vi "Actor Core.vi"(8 "error in":errorcluster, 11 "Display Panel V3 in":refnum<class "Display Panel V3.lvclass">) -> (0 "error out":errorcluster, 3 "Actor out":refnum<class "Actor.lvclass">)   [LabVIEW 2014, in "Display Panel.lvlib" / "Display Panel V3.lvclass"]
doc: "(<B>Filename</B>: Actor Framework.lvlib:Actor.lvclass:Actor Core.vi)\n\nReceives messages to the actor, reacts to them, and initiates any error handling that may shut the actor down.\n\nDescendant classes may override this VI to append parallel tasks for the actor to complete while it handles messages. Overrides use the Call Parent Method node."
uses:
  Display Panel V3.lvclass
  <vilib>/ActorFramework/Actor/Actor.lvclass
  Controls/Numeric Indicator.ctl
  <vilib>/ActorFramework/Actor/Actor.lvclass/Actor.ctl
  <vilib>/ActorFramework/Message Enqueuer/Message Enqueuer.lvclass/Message Enqueuer.ctl
  <vilib>/ActorFramework/Stop Msg/Stop Msg.lvclass/Stop Msg.ctl
  <vilib>/ActorFramework/Message Enqueuer/Init from Existing Queue.vi
  <vilib>/ActorFramework/Message Enqueuer/Enqueue Critical.vi
  <vilib>/express/express shared/transition.llb/Dynamic To Waveform Array.vi
  <vilib>/ActorFramework/Message Priority Queue/Priority Enqueue.vi
  <vilib>/ActorFramework/Message Enqueuer/Message Enqueuer.lvclass
  <vilib>/express/express signal manip/GetorSetDDTAttributes/Get DDT Attributes/Get DDT Properties.xnode
  <vilib>/ActorFramework/Stop Msg/Stop Msg.lvclass
  Generic Instrument/Generic Instrument.lvclass
panel:
  out "String":string
  out "Card #":dbl
  out "Numeric Control":i32
  in  "Waveform Chart":dynamicdata(graph)
  out "Array":T1[](array[typedef])
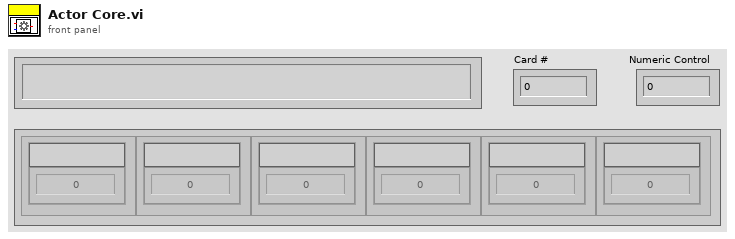
[diagram p1: front panel]
types:
  T1 = typedef "Numeric Indicator.ctl" = cluster{"Numeric Indicator 2":dbl, "String":string}
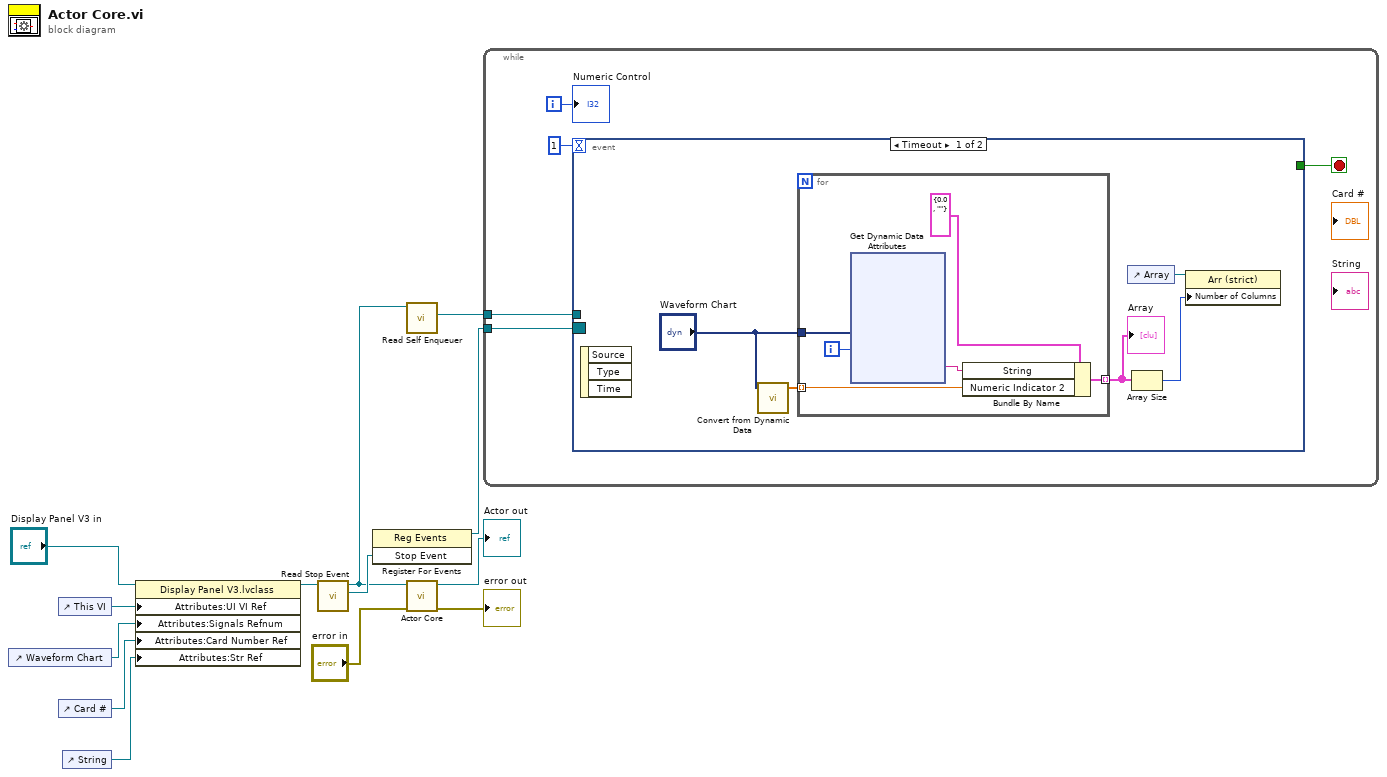
[diagram p0: block diagram]
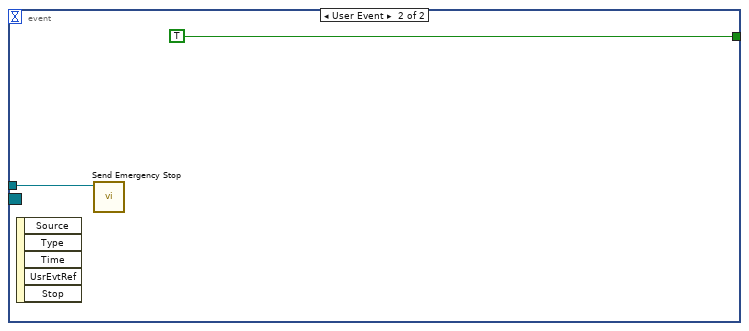
[diagram p2: hidden frame]
diagram:
  n1 = control-ref of="Waveform Chart"() -> (w9:refnum<vi>)
  n2 = control-ref of="This VI"() -> (w10:refnum<vi>)
  n3 = control-ref of="Card #"() -> (w6:refnum<vi>)
  n4 = control-ref of="String"() -> (w5:refnum<vi>)
  n5 = property class="Display Panel V3.lvclass"(reference="Display Panel V3 in", "Attributes:UI VI Ref"=w10, "Attributes:Signals Refnum"=w9, "Attributes:Card Number Ref"=w6, "Attributes:Str Ref"=w5) -> (reference out=w4:refnum<class "Display Panel V3.lvclass">)  [unwired: 1 in, 1 out]
  n6 = call-dynamic "Read Stop Event.vi"("Generic Instrument in"=w4) -> ("Stop Event"=w3:refnum<user-event>, "Generic Instrument out"=w2:refnum<class "Display Panel V3.lvclass">)  [unwired: 8 in, 1 out]
  n7 = register-events(w3) -> (reference out=w7:refnum<event-registration>)  [unwired: 2 in, 1 out]
  n8 = call <vilib>:"Read Self Enqueuer.vi"("Actor"=w2) -> ("Self Enqueuer"=w1:refnum<class "Message Enqueuer.lvclass">)  [unwired: 10 in]
  n9 = call-parent "Actor Core.vi"("error in"="error in", "Actor in"=w2) -> ("error out"=→"error out":errorcluster, "Actor out"=→"Actor out":refnum<class "Actor.lvclass">)  [unwired: 8 in]
  n10 = while {
    tunnel: w7 -> [w18]
    tunnel: w1 -> [w14]
    i -> [w15]
    stop <- w16 stop-if-true
    n11 = event shown="[0] Timeout" {
      selector: w18 -> [_ _]
      dyn-events: _ -> [_ _]
      timeout: 1 -> [_ _]
      tunnel: [_ TRUE] -> w16
      tunnel: w14 -> [_ w39]
      event Timeout {
        n12 = event-data() -> ()  [unwired: 1 in, 3 out]
        n13 = call "Convert from Dynamic Data"("Dynamic Data Type"="Waveform Chart") -> ("Array"=w23:dbl[])  [unwired: 3 in]
        n14 = for {
          tunnel: w23 -> [w28] mode=indexing
          tunnel: "Waveform Chart" -> [w27]
          tunnel: [w25] -> w20 mode=indexing
          i -> [w24]
          n15 = xnode "Get Dynamic Data Attributes"("Signals In"=w27, "Signal Index"=w24) -> ("Signal Name"=w26:string)  [unwired: 1 in, 2 out]
          n16 = Bundle By Name(cluster=T1 {"Numeric Indicator 2"=0.0, "String"=""} ("Cluster 2"), "String"=w26, "Numeric Indicator 2"=w28) -> (w25:T1)
        }
        "Array" <- w20
        n17 = control-ref of="Array"() -> (w21:refnum<vi>)
        n18 = Array Size(array=w20) -> (size(s)=w19:i32)
        n19 = property class="Arr (strict)"(reference=w21, "Number of Columns"=w19) -> ()  [unwired: 1 in, 2 out]
      }
      event User Event {
        n20 = event-data() -> ()  [unwired: 1 in, 5 out]
        n21 = call <vilib>:"Send Emergency Stop.vi"("Message Enqueuer"=w39) -> ()  [unwired: 10 in, 1 out]
      }
    }
    "Numeric Control" <- w15
  }
